vi "Rotation2d_GetRadians.vi"(11 "in ROTATION":T1={"VALUE"=0.0, "COS"=1.0, "SIN"=0.0} {"SIN" format="%13.4f"; "COS" format="%13.4f"; "VALUE" format="%13.4f"}) -> (3 "AngleRadians":dbl)   [LabVIEW 2019, in "Trajectory_Library.lvlib"]
doc: "Get the angle in radians from the rotation.\n\nParameters:\n- ROTATION - The rotation data structure\n\nResults:\n- Angle in radians."
uses:
  Trajectory_Library.lvlib
  TypeDef/ROTATION2D.ctl
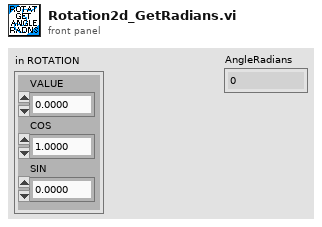
[diagram p1: front panel]
types:
  T1 = typedef "Trajectory_Library.lvlib/ROTATION2D.ctl" = cluster{"VALUE":dbl, "COS":dbl, "SIN":dbl}
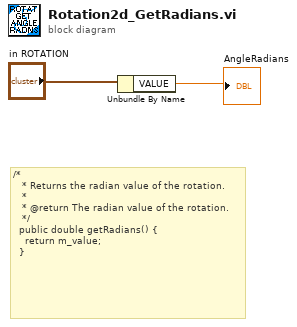
[diagram p0: block diagram]
diagram:
  # "/*\n   * Returns the radian value of the rotation.\n   *\n   * @return The radian value of the rotation.\n   */\n  public double getRadians() {\n    return m_value;\n  }"
  n1 = Unbundle By Name("in ROTATION") -> ("VALUE"=→"AngleRadians":dbl)
